vi "Basic Write.vi"() -> ()   [LabVIEW 2016]
uses:
  <vilib>/Utility/error.llb/DialogType.ctl
  <vilib>/pximc/Initialize Writer Session (DBL).vi
  <vilib>/pximc/Connect (DBL).vi
  <vilib>/pximc/Write (DBL).vi
  <vilib>/pximc/nipximc.lvlib
  <vilib>/measure/NI_MABase.lvlib
panel:
  in  "Connection ID 2":u16=2
  in  "Connection Timeout (s) 2":dbl=60.0 caption="timeout in seconds (-1)"
  in  "Writer Interface 2":tag="PXIMC1" caption="interface"
  in  "Stop Button 2":bool
  out "Samples Written 2":u64=492000000 caption="number of elements written"
  in  "Sample Rate 2":dbl=99900.0
  in  "Samples per Write 2":dbl=100000.0
  in  "Sine Wave Frequency 2":dbl=10.0
  in  "Stop Button":bool
  out "Samples Written":u64=492000000 caption="number of elements written"
  in  "Sample Rate":dbl=99900.0
  in  "Samples per Write":dbl=100000.0
  in  "Sine Wave Frequency":dbl=10.0
  in  "Writer Interface":tag="PXIMC1" caption="interface"
  in  "Connection Timeout (s)":dbl=60.0 caption="timeout in seconds (-1)"
  in  "Connection ID":u16=1
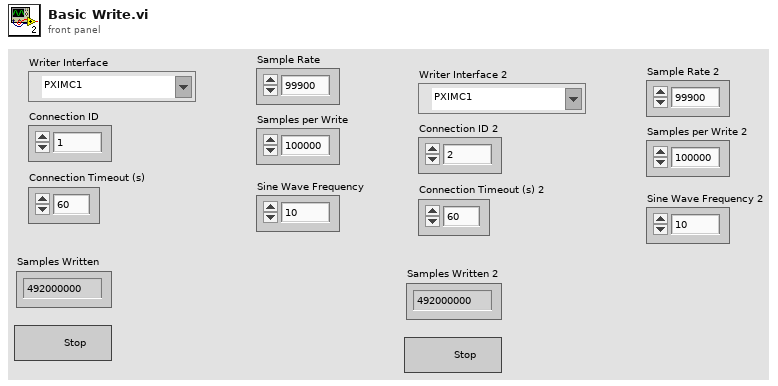
[diagram p1: front panel]
types:
  T1 = typedef "DialogType.ctl" = u16
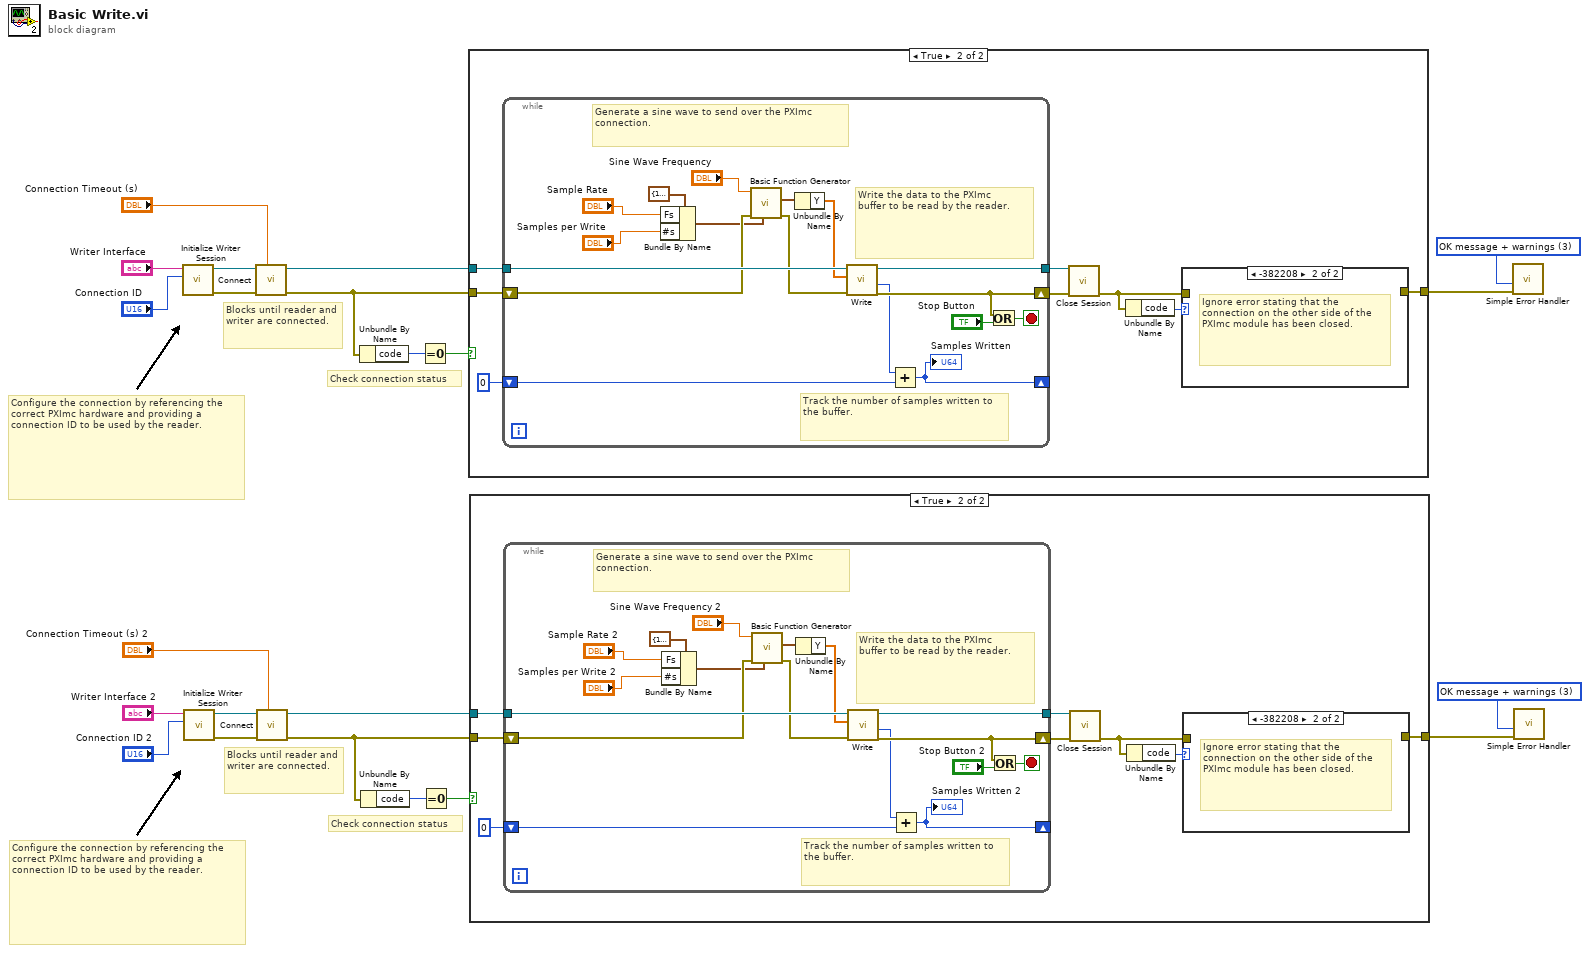
[diagram p0: block diagram]
diagram:
  w11 = T1 3 items=["no dialog", "OK message", "continue or stop message", "OK message + warnings", "continue/stop + warnings"] ("type of dialog (OK msg:1)")
  w12 = T1 3 items=["no dialog", "OK message", "continue or stop message", "OK message + warnings", "continue/stop + warnings"] ("type of dialog (OK msg:1)")
  # "Check connection status"
  # "Blocks until reader and \nwriter are connected."
  # "Configure the connection by referencing the correct PXImc hardware and providing a  connection ID to be used by the reader."
  # "Check connection status"
  # "Blocks until reader and \nwriter are connected."
  # "Configure the connection by referencing the correct PXImc hardware and providing a  connection ID to be used by the reader."
  n1 = call-poly <vilib>:"Initialize Writer Session.vi"("connection id (1)"="Connection ID", "interface"="Writer Interface") -> ("error out"=w21:errorcluster, "session out"=w20:refnum<k21>)  [unwired: 8 in]
  n2 = call-poly <vilib>:"Initialize Writer Session.vi"("connection id (1)"="Connection ID 2", "interface"="Writer Interface 2") -> ("error out"=w2:errorcluster, "session out"=w3:refnum<k21>)  [unwired: 8 in]
  n3 = call-poly <vilib>:"Connect.vi"("timeout in seconds (-1)"="Connection Timeout (s)", "error in (no error)"=w21, "session in"=w20) -> ("error out"=w13:errorcluster, "session out"=w18:refnum<k21>)  [unwired: 7 in]
  n4 = call-poly <vilib>:"Connect.vi"("timeout in seconds (-1)"="Connection Timeout (s) 2", "error in (no error)"=w2, "session in"=w3) -> ("error out"=w10:errorcluster, "session out"=w5:refnum<k21>)  [unwired: 7 in]
  n5 = Unbundle By Name(w13) -> ("code"=w15:i32)
  n6 = Unbundle By Name(w10) -> ("code"=w8:i32)
  n7 = Equal To 0?(x=w15) -> (x = 0?=w14:bool)
  n8 = Equal To 0?(x=w8) -> (x = 0?=w9:bool)
  n9 = case shown="True" w14 {
    tunnel: w18 -> [_ w31]
    tunnel: w13 -> [w23 w30]
    tunnel: [w23 w24] -> w16
    frame False {
      # "The connection was not successful for some reason."
    }
    frame True {
      n10 = while {
        tunnel: w31 -> [w49]
        tunnel: [w48] -> w28
        shift-right: [w43] -> _
        shift-left: u64 0 -> [w44]
        shift-right: [w46] -> w29
        shift-left: w30 -> [w41]
        stop <- w47 stop-if-true
        # "Generate a sine wave to send over the PXImc connection."
        # "Track the number of samples written to the buffer."
        # "Write the data to the PXImc \nbuffer to be read by the reader."
        n11 = Bundle By Name(cluster=cluster{"Fs":dbl, "#s":dbl} {"Fs"=1000.0, "#s"=1000.0} ("sampling info"), "Fs"="Sample Rate", "#s"="Samples per Write") -> (w38:cluster{"Fs":dbl, "#s":dbl})
        n12 = call <vilib>:"Basic Function Generator.vi"("sampling info"=w38, "error in (no error)"=w41, "frequency"="Sine Wave Frequency") -> ("error out"=w34:errorcluster, "signal out"=w35:waveform(dbl))  [unwired: 6 in, 1 out]
        n13 = Unbundle By Name(w35) -> ("Y"=w33:dbl[])
        n14 = call-poly <vilib>:"Write.vi"("error in (no error)"=w34, "data"=w33, "session in"=w49) -> ("error out"=w46:errorcluster, "number of elements written"=w40:u32, "session out"=w48:refnum<k21>)  [unwired: 6 in]
        n15 = Add(x=w40, y=w44) -> (x+y=w43:u64)
        "Samples Written" <- w43
        n16 = Or(x=w46, y="Stop Button") -> (x .or. y?=w47:bool)
      }
      n17 = call <vilib>:"Close Session.vi"("error in (no error)"=w29, "session in"=w28) -> ("error out"=w25:errorcluster)  [unwired: 9 in]
      n18 = Unbundle By Name(w25) -> ("code"=w26:i32)
      n19 = case shown="-382208" w26 {
        tunnel: w25 -> [w32 _]
        tunnel: [w32 _] -> w24
        frame 0, Default {
        }
        frame -382208 {
          # "Ignore error stating that the connection on the other side of the PXImc module has been closed."
        }
      }
    }
  }
  n20 = case shown="True" w9 {
    tunnel: w5 -> [_ w58]
    tunnel: w10 -> [w50 w57]
    tunnel: [w50 w51] -> w7
    frame False {
      # "The connection was not successful for some reason."
    }
    frame True {
      n21 = while {
        tunnel: w58 -> [w76]
        tunnel: [w75] -> w55
        shift-right: [w70] -> _
        shift-left: u64 0 -> [w71]
        shift-right: [w73] -> w56
        shift-left: w57 -> [w68]
        stop <- w74 stop-if-true
        # "Generate a sine wave to send over the PXImc connection."
        # "Track the number of samples written to the buffer."
        # "Write the data to the PXImc \nbuffer to be read by the reader."
        n22 = Bundle By Name(cluster=cluster{"Fs":dbl, "#s":dbl} {"Fs"=1000.0, "#s"=1000.0} ("sampling info"), "Fs"="Sample Rate 2", "#s"="Samples per Write 2") -> (w65:cluster{"Fs":dbl, "#s":dbl})
        n23 = call <vilib>:"Basic Function Generator.vi"("sampling info"=w65, "error in (no error)"=w68, "frequency"="Sine Wave Frequency 2") -> ("error out"=w61:errorcluster, "signal out"=w62:waveform(dbl))  [unwired: 6 in, 1 out]
        n24 = Unbundle By Name(w62) -> ("Y"=w60:dbl[])
        n25 = call-poly <vilib>:"Write.vi"("error in (no error)"=w61, "data"=w60, "session in"=w76) -> ("error out"=w73:errorcluster, "number of elements written"=w67:u32, "session out"=w75:refnum<k21>)  [unwired: 6 in]
        n26 = Add(x=w67, y=w71) -> (x+y=w70:u64)
        "Samples Written 2" <- w70
        n27 = Or(x=w73, y="Stop Button 2") -> (x .or. y?=w74:bool)
      }
      n28 = call <vilib>:"Close Session.vi"("error in (no error)"=w56, "session in"=w55) -> ("error out"=w52:errorcluster)  [unwired: 9 in]
      n29 = Unbundle By Name(w52) -> ("code"=w53:i32)
      n30 = case shown="-382208" w53 {
        tunnel: w52 -> [w59 _]
        tunnel: [w59 _] -> w51
        frame 0, Default {
        }
        frame -382208 {
          # "Ignore error stating that the connection on the other side of the PXImc module has been closed."
        }
      }
    }
  }
  n31 = call <vilib>:"Simple Error Handler.vi"("type of dialog (OK msg:1)"=w12, "error in (no error)"=w16) -> ()  [unwired: 3 in, 5 out]
  n32 = call <vilib>:"Simple Error Handler.vi"("type of dialog (OK msg:1)"=w11, "error in (no error)"=w7) -> ()  [unwired: 3 in, 5 out]
